vi "AddLogPacket (SubVI).vi"(11 "UNDT_Cluster":T1 {"Gain Coeff" format="%#_6e"; "Reserve 1" format="%02x"; "Mux TX/RX" format="%02x"; "ScanDelay" format="%02x"; "PacketCounter" format="%08x"; "SamplingInterval" format="%#_6e"; "Lose Packet" format="%08x"; "EncodersParam2" format="%016x"; "EncodersParam1" format="%016x"; "CRC 8" format="%02x"; "N chanel" format="%02x"; "N tick" format="%02x"; "Ncycle" format="%04x"; "FrameFormatVersion" format="%02x"; "MagicWord" format="%.0x"}) -> ()   [LabVIEW 2017]
uses:
  Control_EU/UNDT_ClusterPackRevers (Type).ctl
  GlobalLog.vi
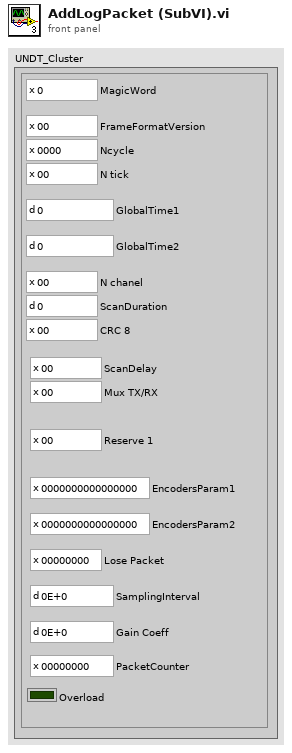
[diagram p1: front panel]
types:
  T1 = typedef "UNDT_ClusterPackRevers (Type).ctl" = cluster{"PacketCounter":u32, "Gain Coeff":sgl, "SamplingInterval":sgl, "Lose Packet":u32, "EncodersParam2":u64, "EncodersParam1":u64, "Reserve 1":u8, "Mux TX/RX":u8, "ScanDelay":u16, "CRC 8":u8, "ScanDuration":u16, "N chanel":u8, "GlobalTime2":u32, "GlobalTime1":u32, "N tick":u8, "Ncycle":u16, "FrameFormatVersion":u8, "MagicWord":u32, "Overload":bool}
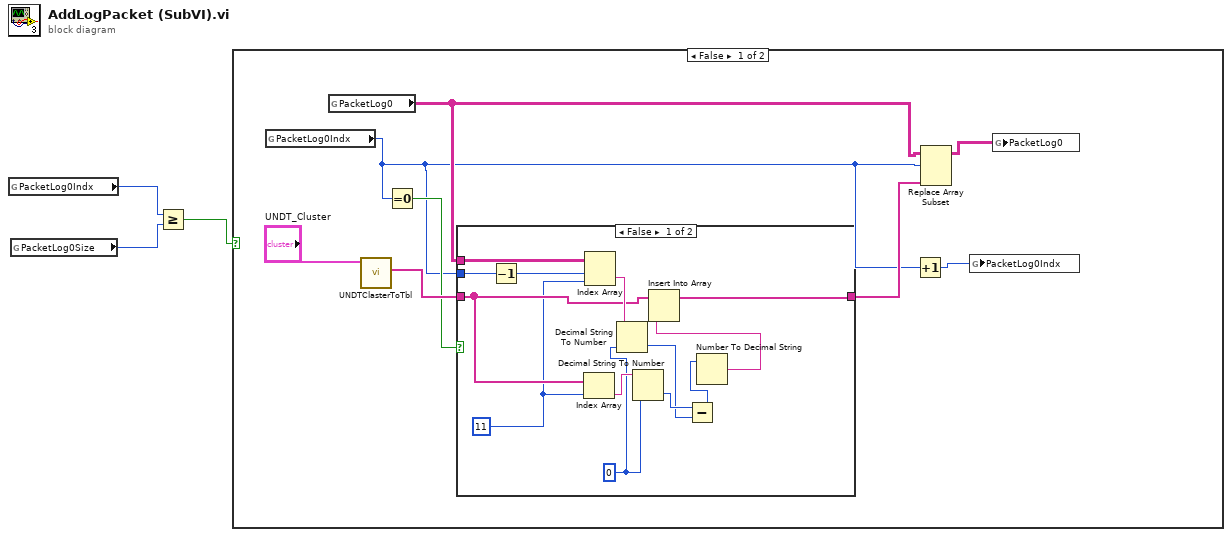
[diagram p0: block diagram]
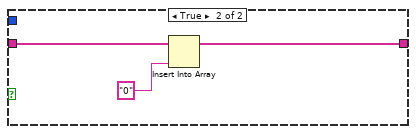
[diagram p2: hidden frame]
diagram:
  n1 = global read "GlobalLog.vi" "PacketLog0Indx"() -> (w3:i32)
  n2 = global read "GlobalLog.vi" "PacketLog0Size"() -> (w2:i32)
  n3 = Greater Or Equal?(x=w3, y=w2) -> (x >= y?=w1:bool)
  n4 = case shown="False" w1 {
    frame False {
      n5 = global read "GlobalLog.vi" "PacketLog0Indx"() -> (w4:i32)
      n6 = global read "GlobalLog.vi" "PacketLog0"() -> (w5:string[][])
      n7 = call "UNDTClasterToTbl.vi"("UNDT_Cluster"="UNDT_Cluster") -> ("appended array"=w8:string[])  [unwired: 9 in, 1 out]
      n8 = Equal To 0?(x=w4) -> (x = 0?=w6:bool)
      n9 = case shown="False" w6 {
        tunnel: w8 -> [w21 w27]
        tunnel: [w23 w25] -> w7
        tunnel: w5 -> [w24 _]
        tunnel: w4 -> [w13 _]
        frame False {
          w18 = i64 0 ("default (0 I32)")
          w20 = 11 ("disabled index (col)")
          n10 = Decrement(x=w13) -> (x-1=w12:i32)
          n11 = Index Array(array=w21, index=w20) -> (element=w19:string)
          n12 = Index Array(array=w24, index (row)=w12, index (col)=w20) -> (element=w22:string)
          n13 = Decimal String To Number(string=w22, default (0L)=w18) -> (number=w16:i64)  [unwired: 1 in, 1 out]
          n14 = Decimal String To Number(string=w19, default (0L)=w18) -> (number=w17:i64)  [unwired: 1 in, 1 out]
          n15 = Subtract(x=w17, y=w16) -> (x-y=w15:i64)
          n16 = Number To Decimal String(number=w15) -> (decimal integer string=w14:string)  [unwired: 1 in]
          n17 = Insert Into Array(array=w21, new element=w14) -> (w23:string[])  [unwired: 1 in]
        }
        frame True {
          n18 = Insert Into Array(array=w27, new element="0" ("new element/subarray")) -> (w25:string[])  [unwired: 1 in]
        }
      }
      n19 = Increment(x=w4) -> (x+1=w11:i32)
      n20 = Replace Array Subset(array=w5, new element=w7, index (row)=w4) -> (w10:string[][])  [unwired: 1 in]
      n21 = global write "GlobalLog.vi" "PacketLog0Indx"(w11) -> ()
      n22 = global write "GlobalLog.vi" "PacketLog0"(w10) -> ()
    }
    frame True {
    }
  }
